vi "DMARS_Euler_Ang2table_Euler_ang (SubVI).vi"(11 "Euler Angles DMARS [º] debug":cluster{"phi":dbl, "theta":dbl, "psi":dbl}) -> (1 "OUTER":dbl, 2 "MIDDLE":dbl, 3 "INNER":dbl)   [LabVIEW 2017]
panel:
  out "Elevation/Azimuth [deg]":dbl[](array[numeric])
  out "Elevation [deg]":dbl
  out "Azimuth [deg]":dbl
  out "Azimuth [rad]":dbl
  out "Elevation [rad]":dbl
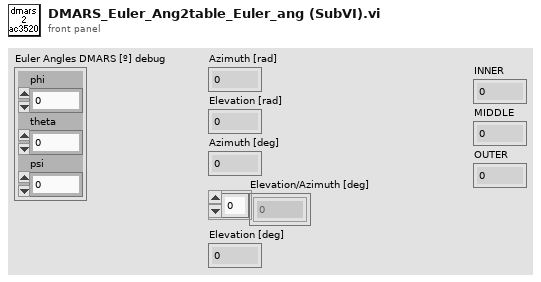
[diagram p1: front panel]
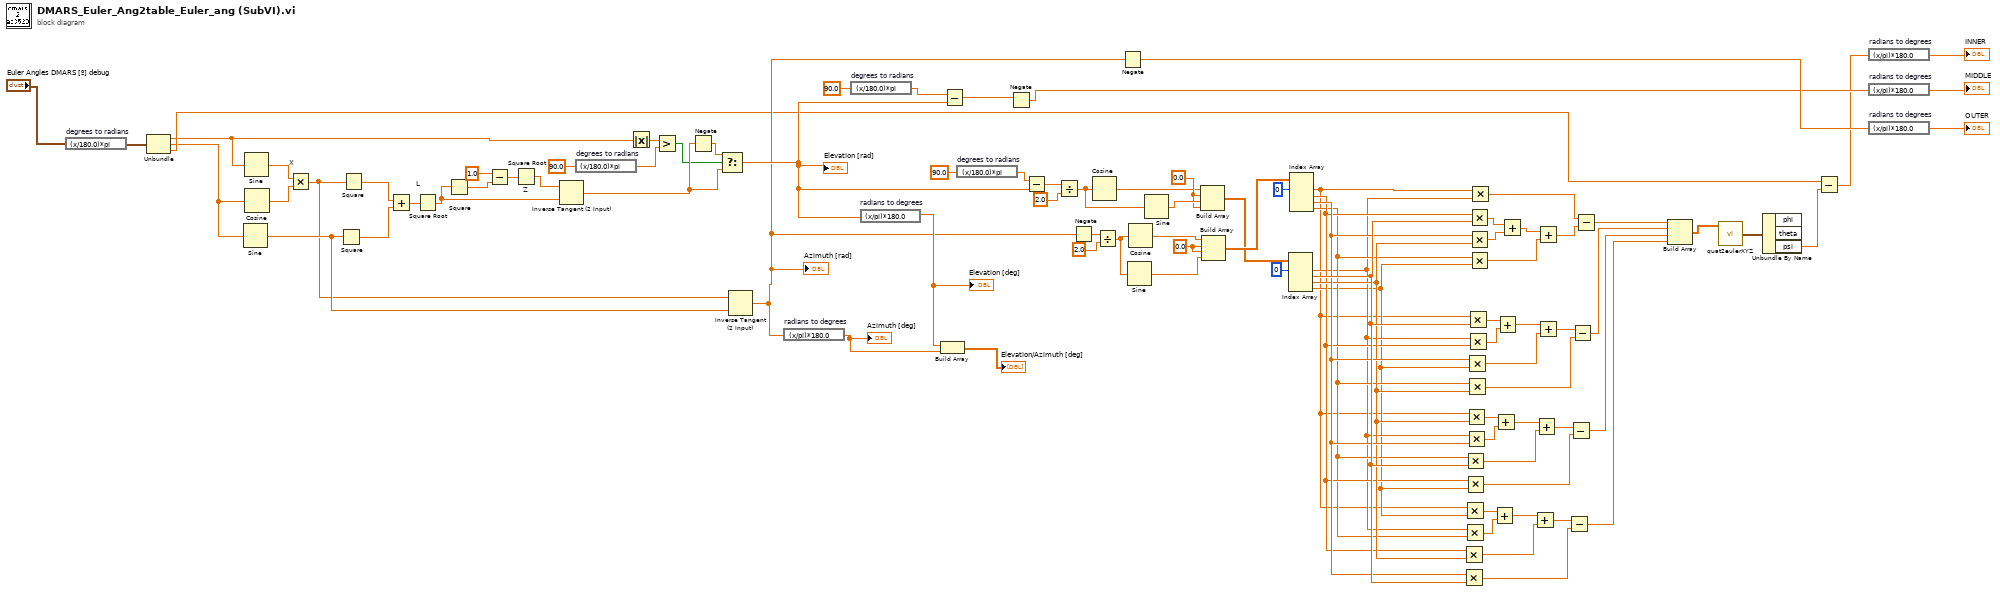
[diagram p0: block diagram]
diagram:
  w28 = 0.0 ("element")
  w21 = 0.0 ("element")
  n1 = expression code="(x/180.0)*pi" "degrees to radians"("Euler Angles DMARS [º] debug") -> (w87:cluster{"phi":dbl, "theta":dbl, "psi":dbl})
  n2 = Unbundle(w87) -> ("phi"=w11:dbl, "theta"=w3:dbl, "psi"=w72:dbl)
  n3 = Sine(x=w3) -> (sin(x)=w18:dbl)
  n4 = Sine(x=w11) -> (sin(x)=w1:dbl)
  n5 = Cosine(x=w3) -> (cos(x)=w2:dbl)
  n6 = Multiply "X"(x=w1, y=w2) -> (x*y=w17:dbl)
  n7 = Square(x=w18) -> (x^2=w5:dbl)
  n8 = Square(x=w17) -> (x^2=w4:dbl)
  n9 = Add(x=w4, y=w5) -> (x+y=w6:dbl)
  n10 = Square Root "L"(x=w6) -> (sqrt(x)=w9:dbl)
  n11 = Square(x=w9) -> (x^2=w7:dbl)
  n12 = Subtract(x=1.0, y=w7) -> (x-y=w80:dbl)
  n13 = Square Root "Z"(x=w80) -> (sqrt(x)=w81:dbl)
  n14 = Inverse Tangent (2 Input)(1:w9, 2:w81) -> (0:w16:dbl)
  n15 = expression code="(x/180.0)*pi" "degrees to radians"(90.0 ("y")) -> (w13:dbl)
  n16 = Absolute Value(x=w11) -> (abs(x)=w12:dbl)
  n17 = Greater?(x=w12, y=w13) -> (0:w14:bool)
  n18 = Negate(x=w16) -> (-x=w15:dbl)
  n19 = Select(t=w15, s=w14, f=w16) -> (s? t:f=w83:dbl)
  "Elevation [rad]" <- w83
  n20 = Inverse Tangent (2 Input)(1:w18, 2:w17) -> (0:w82:dbl)
  "Azimuth [rad]" <- w82
  n21 = expression code="(x/pi)*180.0" "radians to degrees"(w82) -> (w85:dbl)
  "Azimuth [deg]" <- w85
  n22 = expression code="(x/180.0)*pi" "degrees to radians"(90.0 ("y")) -> (w78:dbl)
  n23 = expression code="(x/pi)*180.0" "radians to degrees"(w83) -> (w84:dbl)
  "Elevation [deg]" <- w84
  n24 = Build Array(w84, w85) -> (→"Elevation/Azimuth [deg]":dbl[])
  n25 = Subtract(x=w78, y=w83) -> (x-y=w79:dbl)
  n26 = expression code="(x/180.0)*pi" "degrees to radians"(90.0 ("y")) -> (w25:dbl)
  n27 = Negate(x=w79) -> (-x=w90:dbl)
  n28 = Subtract(x=w25, y=w83) -> (x-y=w74:dbl)
  n29 = Divide(x=w74, y=2.0) -> (x/y=w30:dbl)
  n30 = Negate(x=w82) -> (-x=w19:dbl)
  n31 = Cosine(x=w30) -> (cos(x)=w27:dbl)
  n32 = Divide(x=w19, y=2.0) -> (x/y=w22:dbl)
  n33 = Negate(x=w82) -> (-x=w92:dbl)
  n34 = Sine(x=w22) -> (sin(x)=w23:dbl)
  n35 = Cosine(x=w22) -> (cos(x)=w29:dbl)
  n36 = Sine(x=w30) -> (sin(x)=w31:dbl)
  n37 = Build Array(w27, w28, w31, w28) -> (w75:dbl[])
  n38 = Build Array(w29, w21, w21, w23) -> (w76:dbl[])
  n39 = Index Array(array=w75, index #1=0 ("index")) -> (element #1=w63:dbl, element #2=w68:dbl, element #3=w66:dbl, element #4=w62:dbl)  [unwired: 3 in]
  n40 = Index Array(array=w76, index #1=0 ("index")) -> (element #1=w61:dbl, element #2=w65:dbl, element #3=w67:dbl, element #4=w64:dbl)  [unwired: 3 in]
  n41 = Multiply(x=w65, y=w66) -> (x*y=w59:dbl)
  n42 = Multiply(x=w67, y=w68) -> (x*y=w60:dbl)
  n43 = Multiply(x=w61, y=w62) -> (x*y=w55:dbl)
  n44 = Multiply(x=w63, y=w64) -> (x*y=w56:dbl)
  n45 = Multiply(x=w64, y=w68) -> (x*y=w49:dbl)
  n46 = Multiply(x=w65, y=w62) -> (x*y=w48:dbl)
  n47 = Multiply(x=w61, y=w66) -> (x*y=w53:dbl)
  n48 = Multiply(x=w63, y=w67) -> (x*y=w52:dbl)
  n49 = Multiply(x=w67, y=w62) -> (x*y=w45:dbl)
  n50 = Multiply(x=w64, y=w66) -> (x*y=w46:dbl)
  n51 = Multiply(x=w61, y=w68) -> (x*y=w41:dbl)
  n52 = Multiply(x=w63, y=w65) -> (x*y=w42:dbl)
  n53 = Multiply(x=w65, y=w68) -> (x*y=w34:dbl)
  n54 = Multiply(x=w67, y=w66) -> (x*y=w35:dbl)
  n55 = Multiply(x=w64, y=w62) -> (x*y=w37:dbl)
  n56 = Multiply(x=w61, y=w63) -> (x*y=w39:dbl)
  n57 = Add(x=w55, y=w56) -> (x+y=w57:dbl)
  n58 = Add(x=w53, y=w52) -> (x+y=w51:dbl)
  n59 = Add(x=w41, y=w42) -> (x+y=w43:dbl)
  n60 = Add(x=w34, y=w35) -> (x+y=w36:dbl)
  n61 = Add(x=w57, y=w59) -> (x+y=w58:dbl)
  n62 = Add(x=w51, y=w49) -> (x+y=w50:dbl)
  n63 = Add(x=w36, y=w37) -> (x+y=w38:dbl)
  n64 = Add(x=w43, y=w45) -> (x+y=w44:dbl)
  n65 = Subtract(x=w58, y=w60) -> (x-y=w69:dbl)
  n66 = Subtract(x=w50, y=w48) -> (x-y=w54:dbl)
  n67 = Subtract(x=w44, y=w46) -> (x-y=w47:dbl)
  n68 = Subtract(x=w39, y=w38) -> (x-y=w40:dbl)
  n69 = Build Array(w40, w47, w54, w69) -> (w70:dbl[])
  n70 = call "quat2eulerXYZ.vi"("Quaternions"=w70) -> ("Euler Angles [rad]"=w71:cluster{"phi":dbl, "theta":dbl, "psi":dbl})  [unwired: 10 in]
  n71 = Unbundle By Name(w71) -> ("psi"=w73:dbl)  [unwired: 2 out]
  n72 = Subtract(x=w72, y=w73) -> (x-y=w88:dbl)
  n73 = expression code="(x/pi)*180.0" "radians to degrees"(w88) -> (→"INNER":dbl)
  n74 = expression code="(x/pi)*180.0" "radians to degrees"(w90) -> (→"MIDDLE":dbl)
  n75 = expression code="(x/pi)*180.0" "radians to degrees"(w92) -> (→"OUTER":dbl)
